vi "ScaleUp_corrSD.vi"(1 "Data":dbl[][](array[numeric]), 2 "ScaleUp":dbl) -> (0 "Data corrected":dbl[][](array[numeric]))   [LabVIEW 2020]
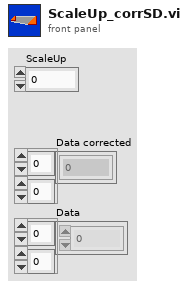
[diagram p1: front panel]
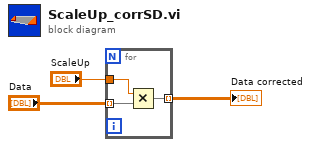
[diagram p0: block diagram]
diagram:
  n1 = for {
    tunnel: "Data" -> [w5] mode=indexing
    tunnel: "ScaleUp" -> [w6]
    tunnel: [w4] -> w1 mode=indexing
    n2 = Multiply(x=w6, y=w5) -> (x*y=w4:dbl[])
  }
  "Data corrected" <- w1
